vi "Get Pixel Format Data From Pointer.vi"(8 "error in (no error)":errorcluster, 11 "Pixel Format Pointer":u32 format="%.0x") -> (0 "error out":errorcluster, 3 "Data":T1 {"Format" format="%.0x"; "Next Pointer" format="%.0x"; "Rmask" format="%.0x"; "Gmask" format="%.0x"; "Bmask" format="%.0x"; "Amask" format="%.0x"; "Palette Pointer" format="%.0x"})   [LabVIEW 2015, in "SDL2 Utility.lvlib"]
uses:
  SDL2 Utility.lvlib
  LibSDL2 Wrapper/Controls/Pixel Formal.ctl
  <vilib>/Utility/importsl/GetValueByPointer/datatype.ctl
  <vilib>/Utility/importsl/GetValueByPointer/GetValueByPointer.xnode
  LibSDL2 Wrapper/LibSDL2.lvlib
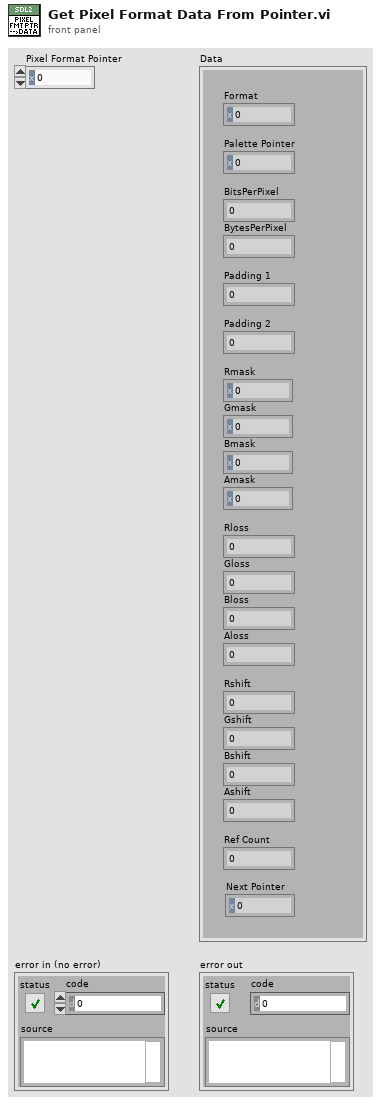
[diagram p1: front panel]
types:
  T1 = typedef "LibSDL2.lvlib/Pixel Formal.ctl" = cluster{"Format":u32, "Palette Pointer":u32, "BitsPerPixel":u8, "BytesPerPixel":u8, "Padding 1":u8, "Padding 2":u8, "Rmask":u32, "Gmask":u32, "Bmask":u32, "Amask":u32, "Rloss":u8, "Gloss":u8, "Bloss":u8, "Aloss":u8, "Rshift":u8, "Gshift":u8, "Bshift":u8, "Ashift":u8, "Ref Count":i32, "Next Pointer":u32}
  T2 = enum32{"pack1", "pack2", "pack4", "pack8", "pack16"}
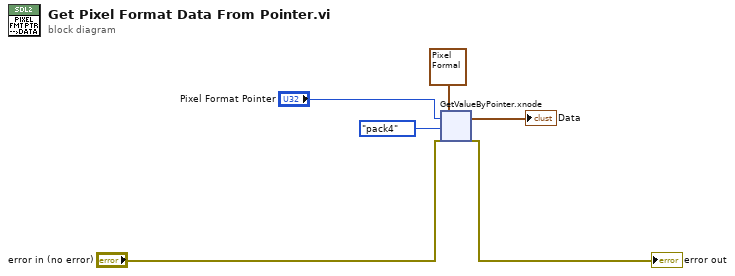
[diagram p0: block diagram]
diagram:
  n1 = xnode "GetValueByPointer.xnode"("Pointer"="Pixel Format Pointer", "InputType"=T1 {"Format"=0, "Palette Pointer"=0, "BitsPerPixel"=0, "BytesPerPixel"=0, "Padding 1"=0, "Padding 2"=0, "Rmask"=0, "Gmask"=0, "Bmask"=0, "Amask"=0, "Rloss"=0, "Gloss"=0, "Bloss"=0, "Aloss"=0, "Rshift"=0, "Gshift"=0, "Bshift"=0, "Ashift"=0, "Ref Count"=0, "Next Pointer"=0} ("Pixel Format"), "PackType"=T2."pack4", "ErrorIn"="error in (no error)") -> ("Output"=→"Data":T1, "ErrorOut"=→"error out":errorcluster)
